vi "TrippLiteUPS_ReadStatus.vi"(8 "ErrorIn":errorcluster, 11 "UPSRefIn":refnum<visa-resource-name>="Port4") -> (0 "ErrorOut":errorcluster, 5 "UPS":T1 {"V" format="%.1f"; "A" format="%.1f"; "Hz" format="%.1f"; "%" format="%.1f"})   [LabVIEW 2018]
uses:
  Controls/Clusts/UPS_Status_Clust.ctl
  <vilib>/Instr/_visa.llb/VISA Configure Serial Port (Instr).vi
panel:
  out "Device":dbl
  out "Status":string
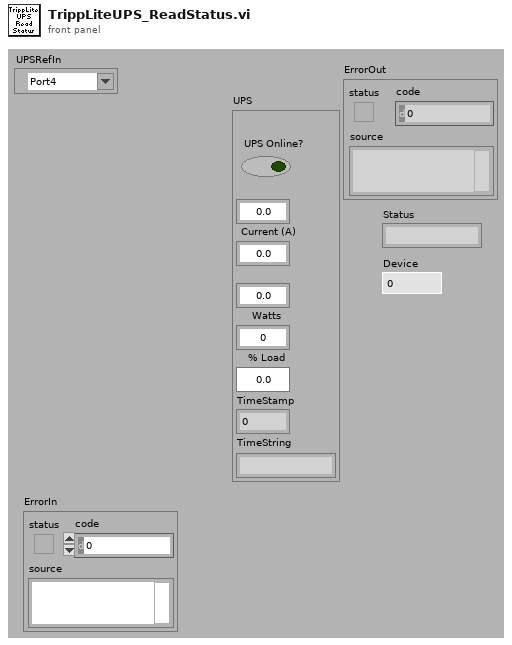
[diagram p1: front panel]
types:
  T1 = typedef "UPS_Status_Clust.ctl" = cluster{"Prsnt?":bool, "V":dbl, "A":dbl, "Hz":dbl, "W":dbl, "%":dbl, "TimeStamp":dbl, "TimeString":string}
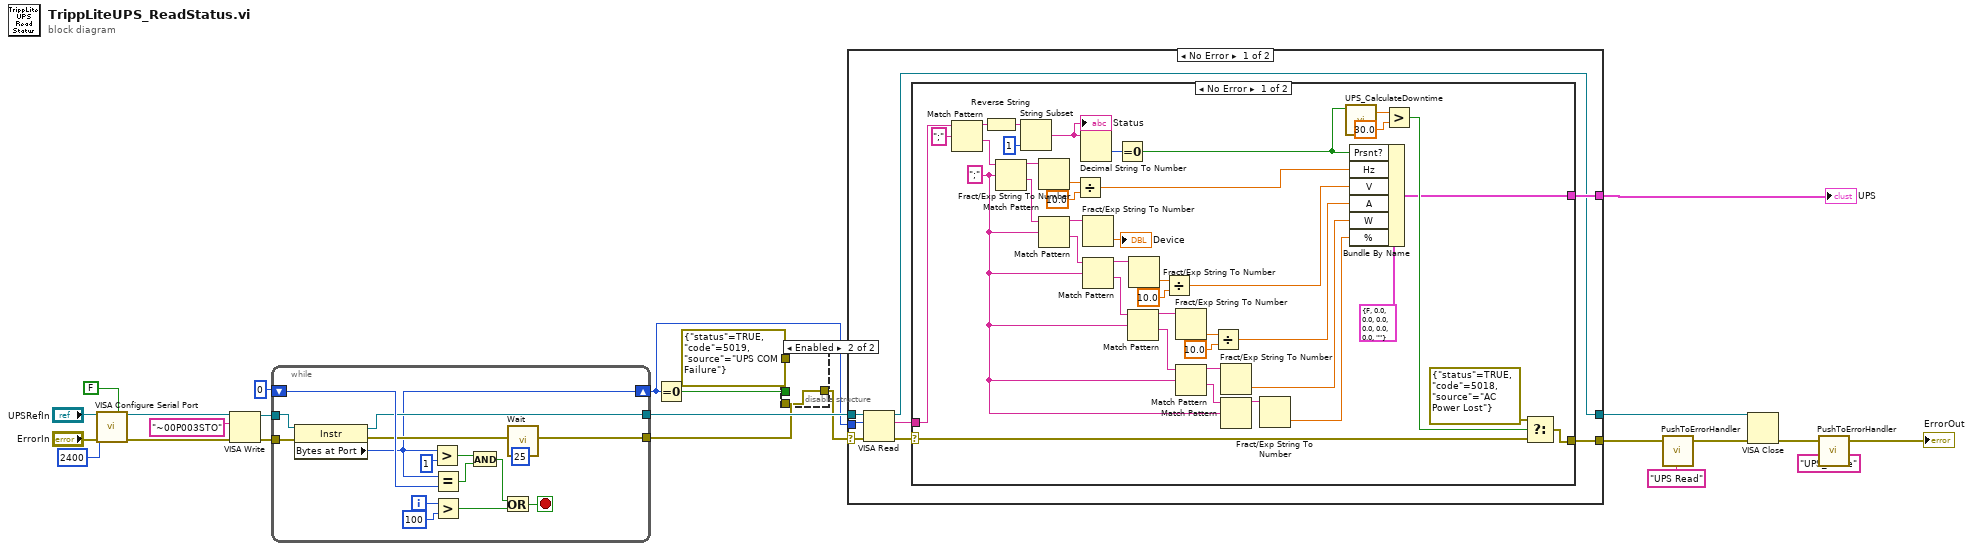
[diagram p0: block diagram]
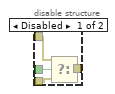
[diagram p2: hidden frame]
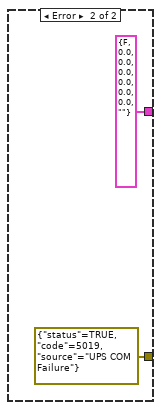
[diagram p3: hidden frame]
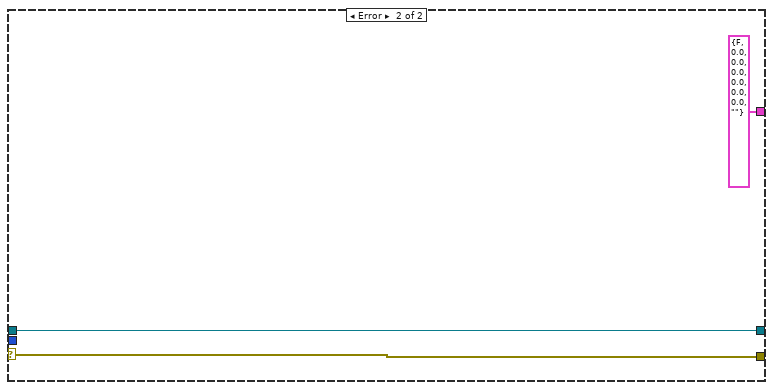
[diagram p4: hidden frame]
diagram:
  n1 = call-poly "VISA Configure Serial Port"("VISA resource name"="UPSRefIn", "Enable Termination\nChar (T)"=FALSE ("Enable Termination\nChar (T)"), "baud rate (9600)"=u32 2400, "error in (no error)"="ErrorIn") -> ("VISA resource name out"=w6:refnum<visa-resource-name>, "error out"=w3:errorcluster)  [unwired: 10 in]
  n2 = VISA Write(VISA resource name=w6, write buffer="~00P003STO", error in (no error)=w3) -> (VISA resource name out=w21:refnum<visa-resource-name>, error out=w19:errorcluster)  [unwired: 1 out]
  n3 = while {
    shift-right: [w28] -> w14
    shift-left: u32 0 ("byte count") -> [w34]
    tunnel: w19 -> [w40]
    tunnel: w21 -> [w39]
    tunnel: [w31] -> w16
    tunnel: [w33] -> w20
    i -> [w38]
    stop <- w36 stop-if-true
    n4 = property class="Instr"(reference=w39, error in=w40) -> (reference out=w33:refnum<visa-resource-name>, error out=w32:errorcluster, "Bytes at Port"=w28:u32)
    n5 = Greater?(x=w28, y=u32 1) -> (0:w26:bool)
    n6 = Equal?(x=w28, y=w34) -> (x = y?=w35:bool)
    n7 = Greater?(x=w38, y=100) -> (0:w25:bool)
    n8 = And(x=w26, y=w35) -> (x .and. y?=w29:bool)
    n9 = Or(x=w29, y=w25) -> (x .or. y?=w36:bool)
    n10 = call "Wait.vi"("Wait (ms)"=u32 25, "ErrorIn"=w32) -> ("ErrorOut"=w31:errorcluster)  [unwired: 9 in]
  }
  n11 = Equal To 0?(x=w14) -> (x = 0?=w18:bool)
  n12 = disable-structure shown="Enabled" {
    disable-tunnel: w18 -> [w44 _]
    disable-tunnel: errorcluster {"status"=TRUE, "code"=5019, "source"="UPS COM Failure"} ("error IO") -> [w43 _]
    disable-tunnel: w16 -> [w42 w45]
    disable-tunnel: [w41 w45] -> w15
    frame Disabled {
      n13 = Select(t=w43, s=w44, f=w42) -> (s? t:f=w41:errorcluster)
    }
    frame Enabled {
    }
  }
  n14 = case shown="No Error" w15 {
    selector: w15 -> [w49 w97]
    tunnel: [w52 T1 {"Prsnt?"=FALSE, "V"=0.0, "A"=0.0, "Hz"=0.0, "W"=0.0, "%"=0.0, "TimeStamp"=0.0, "TimeString"=""} ("UPS")] -> w23
    tunnel: [w46 w99] -> w10
    tunnel: w20 -> [w51 w99]
    tunnel: w14 -> [w50 _]
    tunnel: [w47 w97] -> w13
    frame No Error {
      n15 = VISA Read(VISA resource name=w51, byte count=w50, error in (no error)=w49) -> (VISA resource name out=w46:refnum<visa-resource-name>, read buffer=w53:string, error out=w48:errorcluster)  [unwired: 1 out]
      n16 = case shown="No Error" w48 {
        selector: w48 -> [w59 _]
        tunnel: w53 -> [w94 _]
        tunnel: [w54 T1 {"Prsnt?"=FALSE, "V"=0.0, "A"=0.0, "Hz"=0.0, "W"=0.0, "%"=0.0, "TimeStamp"=0.0, "TimeString"=""} ("UPS")] -> w52
        tunnel: [w58 errorcluster {"status"=TRUE, "code"=5019, "source"="UPS COM Failure"} ("error IO")] -> w47
        frame No Error {
          w86 = ";" ("regular expression")
          n17 = Match Pattern(string=w94, regular expression=";") -> (before substring=w92:string, after substring=w89:string)  [unwired: 1 in, 2 out]
          n18 = Reverse String(1:w92) -> (0:w91:string)
          n19 = Match Pattern(string=w89, regular expression=w86) -> (before substring=w81:string, after substring=w88:string)  [unwired: 1 in, 2 out]
          n20 = String Subset(string=w91, length (rest)=1 ("length (rest)")) -> (substring=w61:string)  [unwired: 1 in]
          "Status" <- w61
          n21 = Fract/Exp String To Number(string=w81) -> (number=w82:dbl)  [unwired: 3 in, 1 out]
          n22 = Match Pattern(string=w88, regular expression=w86) -> (before substring=w75:string, after substring=w85:string)  [unwired: 1 in, 2 out]
          n23 = Divide(x=w82, y=10.0) -> (x/y=w68:dbl)
          n24 = Decimal String To Number(string=w61) -> (number=w69:i32)  [unwired: 2 in, 1 out]
          n25 = Fract/Exp String To Number(string=w75) -> (number=→"Device":dbl)  [unwired: 3 in, 1 out]
          n26 = Match Pattern(string=w85, regular expression=w86) -> (before substring=w74:string, after substring=w84:string)  [unwired: 1 in, 2 out]
          n27 = Equal To 0?(x=w69) -> (x = 0?=w60:bool)
          n28 = Match Pattern(string=w84, regular expression=w86) -> (before substring=w73:string, after substring=w83:string)  [unwired: 1 in, 2 out]
          n29 = Fract/Exp String To Number(string=w74) -> (number=w79:dbl)  [unwired: 3 in, 1 out]
          n30 = Divide(x=w79, y=10.0) -> (x/y=w57:dbl)
          n31 = Fract/Exp String To Number(string=w73) -> (number=w76:dbl)  [unwired: 3 in, 1 out]
          n32 = Match Pattern(string=w83, regular expression=w86) -> (before substring=w72:string, after substring=w87:string)  [unwired: 1 in, 2 out]
          n33 = Divide(x=w76, y=10.0) -> (x/y=w56:dbl)
          n34 = Fract/Exp String To Number(string=w72) -> (number=w67:dbl)  [unwired: 3 in, 1 out]
          n35 = Match Pattern(string=w87, regular expression=w86) -> (before substring=w71:string)  [unwired: 1 in, 3 out]
          n36 = Fract/Exp String To Number(string=w71) -> (number=w66:dbl)  [unwired: 3 in, 1 out]
          n37 = call "UPS_CalculateDowntime.vi"("Prsnt?"=w60) -> ("Downtime(s)"=w65:dbl)  [unwired: 4 in]
          n38 = Bundle By Name(cluster=T1 {"Prsnt?"=FALSE, "V"=0.0, "A"=0.0, "Hz"=0.0, "W"=0.0, "%"=0.0, "TimeStamp"=0.0, "TimeString"=""} ("UPS"), "Prsnt?"=w60, "Hz"=w68, "V"=w57, "A"=w56, "W"=w67, "%"=w66) -> (w54:T1)
          n39 = Greater?(x=w65, y=30.0) -> (0:w63:bool)
          n40 = Select(t=errorcluster {"status"=TRUE, "code"=5018, "source"="AC Power Lost"} ("error IO"), s=w63, f=w59) -> (s? t:f=w58:errorcluster)
        }
        frame Error {
        }
      }
    }
    frame Error {
    }
  }
  "UPS" <- w23
  n41 = call "PushToErrorHandler.vi"("ErrorIn"=w13, "ErrorLocation"="UPS Read") -> ("ErrorOut"=w11:errorcluster)  [unwired: 5 in]
  n42 = VISA Close(VISA resource name=w10, error in (no error)=w11) -> (error out=w9:errorcluster)
  n43 = call "PushToErrorHandler.vi"("ErrorIn"=w9, "ErrorLocation"="UPS_Close") -> ("ErrorOut"=→"ErrorOut":errorcluster)  [unwired: 5 in]
